vi "dfd_Convert Filter to String.vi"(5 "indent order":i32, 7 "format string":string="%-+022.16e", 11 "filter":T1={"mSRate_Fs"=1.0, "mSRate_Version"="1.0", "mSRate_Comments"="", "mSRate_OrgCoef"={"type"=enum."Undefined", "gain"=1.0, "coef a (k)"=[], "coef b (v)"=[]}, "mSRate_CurCoef"={"type"=enum."Undefined", "gain"=1.0, "coef a (k)"=[], "coef b (v)"=[]}, "mSRate_Quantized?"=FALSE, "mSRate_QCoef"={"type"=enum."Undefined", "gain"=1.0, "coef a (k)"=[], "coef b (v)"=[]}, "mSRate_QSettings"=[], "mSRate_Order"=0, "mSRate_Scaling"={"mSRate_ScaleByPowerOf2?"=FALSE, "mSRate_ScaleType"=enum."No Norm"}} {"mSRate_QSettings"."source" items=["Coef a/k"=0, "Coef b/v"=7, "Input"=1, "Output"=2, "Multiplicand"=3, "Product"=4, "Sum"=5, "Delay"=6, "Gain"=8]}) -> (3 "xml string":string)   [LabVIEW 2017, in "NI_DigFilter_Process.lvlib"]
uses:
  <vilib>/addons/Digital Filter Design/NI_DigFilter_Process.lvlib
  <vilib>/addons/Digital Filter Design/_Objects.llb/DFD Filter Obj.ctl
  <vilib>/addons/Digital Filter Design/_Objects.llb/DFD Filter Coef.ctl
  <vilib>/addons/Digital Filter Design/_Objects.llb/DFD Filter Structure Type Selector.ctl
  <vilib>/addons/Digital Filter Design/_Objects.llb/dfd_Internal Quantization Settings.ctl
  <vilib>/addons/Digital Filter Design/_Objects.llb/dfd_Internal Quantization Srcs.ctl
  <vilib>/addons/Digital Filter Design/_Objects.llb/DFD Coef Norm Type.ctl
  <vilib>/addons/Digital Filter Design/NI_DigFilterLicensed.lvlib
panel:
  in  "ZPK format string":string="%.16e"
  out "error out":errorcluster
  in  "error in (no error)":errorcluster
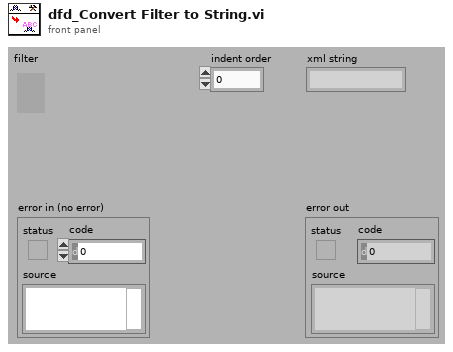
[diagram p1: front panel]
types:
  T1 = typedef "NI_DigFilterLicensed.lvlib/DFD Filter Obj.ctl" = cluster{"mSRate_Fs":dbl, "mSRate_Version":string, "mSRate_Comments":string, "mSRate_OrgCoef":T2, "mSRate_CurCoef":T2, "mSRate_Quantized?":bool, "mSRate_QCoef":T2, "mSRate_QSettings":T4[], "mSRate_Order":i32, "mSRate_Scaling":cluster{"mSRate_ScaleByPowerOf2?":bool, "mSRate_ScaleType":T6}}
  T2 = typedef "NI_DigFilterLicensed.lvlib/DFD Filter Coef.ctl" = cluster{"type":T3, "gain":dbl, "coef a (k)":dbl[], "coef b (v)":dbl[]}
  T3 = typedef "NI_DigFilterLicensed.lvlib/DFD Filter Structure Type Selector.ctl" = enum16{"Undefined", "FIR Direct Form", "FIR Direct Form Transposed", "FIR Symmetric", "FIR Antisymmetric", "IIR Direct Form I", "IIR Direct Form I Transposed", "IIR Direct Form II", "IIR Direct Form II Transposed", "IIR Cascaded Second Order Sections Form I", "IIR Cascaded Second Order Sections Form I Transposed", "IIR Cascaded Second Order Sections Form II", "IIR Cascaded Second Order Sections Form II Transposed", "Lattice Allpass (basic sections)", "Lattice Allpass (one multiplier sections)", "Lattice Allpass (normalized sections)", "Lattice AR (basic sections)", "Lattice AR (one multiplier sections)", "Lattice AR (normalized sections)", "Lattice MA (minimum phase)", "Lattice MA (maximum phase)", "Lattice ARMA (basic sections)", "Lattice ARMA (one multiplier sections)", "Lattice ARMA (normalized sections)"}
  T4 = typedef "NI_DigFilterLicensed.lvlib/dfd_Internal Quantization Settings.ctl" = cluster{"source":T5, "wl":i16, "iwl":i16, "overflow mode":enum16{"Saturation", "Wrap"}, "rounding mode":enum16{"Nearest", "Truncation"}, "signed?":bool}
  T5 = typedef "NI_DigFilterLicensed.lvlib/dfd_Internal Quantization Srcs.ctl" = u16
  T6 = typedef "NI_DigFilterLicensed.lvlib/DFD Coef Norm Type.ctl" = enum16{"No Norm", "Time Domain 1-Norm", "Time Domain 2-Norm", "Time Domain Inf-Norm"}
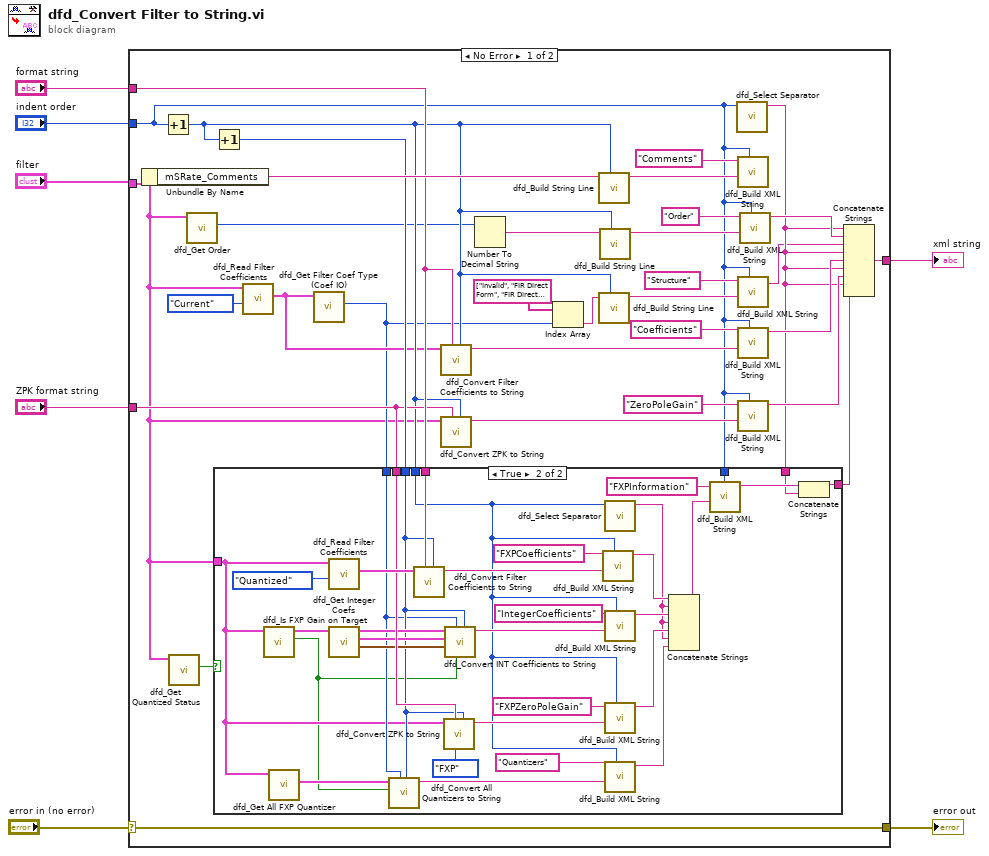
[diagram p0: block diagram]
diagram:
  n1 = case shown="No Error" "error in (no error)" {
    selector: "error in (no error)" -> [w31 w75]
    tunnel: "filter" -> [w10 _]
    tunnel: "format string" -> [w24 _]
    tunnel: [w32 _] -> w6
    tunnel: [w31 w75] -> w5
    tunnel: "indent order" -> [w16 _]
    tunnel: "ZPK format string" -> [w23 _]
    frame No Error {
      n2 = Unbundle By Name(w10) -> ("mSRate_Comments"=w29:string)
      n3 = Increment(x=w16) -> (x+1=w19:i32)
      n4 = call <vilib>:"dfd_Get Quantized Status.vi"("filter in"=w10) -> ("quantized?"=w26:bool)  [unwired: 1 in, 9 out]
      n5 = call <vilib>:"dfd_Get Order.vi"("filter in"=w10) -> ("order"=w11:i32)  [unwired: 1 in, 9 out]
      n6 = Increment(x=w19) -> (x+1=w25:i32)
      n7 = call <vilib>:"dfd_Read Filter Coefficients.vi"("coef source"=enum16{"Original", "Current", "Quantized"}."Current", "filter in"=w10) -> ("filter coef"=w14:T2)  [unwired: 1 in, 8 out]
      n8 = call <vilib>:"dfd_Get Filter Coef Type (Coef IO).vi"("filter coef in"=w14) -> ("type"=w12:T3)  [unwired: 1 in, 9 out]
      n9 = call <vilib>:"dfd_Convert Filter Coefficients to String.vi"("indent order"=w19, "format string"=w24, "filter coef"=w14) -> ("xml string out"=w38:string)  [unwired: 2 in, 6 out]
      n10 = call <vilib>:"dfd_Convert ZPK to String.vi"("indent order"=w19, "format string"=w23, "filter"=w10) -> ("xml string"=w30:string)  [unwired: 3 in, 5 out]
      n11 = Number To Decimal String(number=w11) -> (decimal integer string=w21:string)  [unwired: 1 out]
      n12 = Index Array(array=string[] ["Invalid", "FIR Direct Form", "FIR Direct Form Transposed", "FIR Symmetric", "FIR Antisymmetric", "IIR Direct Form I", "IIR Direct Form I Transposed", "IIR Direct Form II", "IIR Direct Form II Transposed", "IIR Cascaded Second-Order Sections Form I", "IIR Cascaded Second-Order Sections Form I Transposed", "IIR Cascaded Second-Order Sections Form II", "IIR Cascaded Second-Order Sections Form II Transposed", "Lattice Allpass (basic sections)", "Lattice Allpass (one multiplier sections)", "Lattice Allpass (normalized sections)", "Lattice AR (basic sections)", "Lattice AR (one multiplier sections)", "Lattice AR (normalized sections)", "Lattice MA (minimum phase)", "Lattice MA (maximum phase)", "Lattice ARMA (basic sections)", "Lattice ARMA (one multiplier sections)", "Lattice ARMA (normalized sections)"] ("Strings []"), index=w12) -> (element=w13:string)
      n13 = call <vilib>:"dfd_Build String Line.vi"("indent order"=w19, "string"=w29) -> ("string line"=w22:string)  [unwired: 9 out]
      n14 = call <vilib>:"dfd_Build String Line.vi"("indent order"=w19, "string"=w13) -> ("string line"=w28:string)  [unwired: 9 out]
      n15 = call <vilib>:"dfd_Build String Line.vi"("indent order"=w19, "string"=w21) -> ("string line"=w20:string)  [unwired: 9 out]
      n16 = call <vilib>:"dfd_Select Separator.vi"("indent order"=w16) -> ("separator"=w15:string)  [unwired: 10 out]
      n17 = case shown="True" w26 {
        tunnel: w10 -> [_ w43]
        tunnel: [_ w53] -> w33
        tunnel: w24 -> [_ w73]
        tunnel: w16 -> [_ w71]
        tunnel: w19 -> [_ w51]
        tunnel: w25 -> [_ w45]
        tunnel: w23 -> [_ w60]
        tunnel: w15 -> [_ w52]
        tunnel: w12 -> [_ w44]
        frame False {
        }
        frame True {
          n18 = call <vilib>:"dfd_Is FXP Gain on Target.vi"("filter in"=w43) -> ("Gain on Target?"=w42:bool, "dup filter out"=w41:T1)  [unwired: 9 out]
          n19 = call <vilib>:"dfd_Get All FXP Quantizer.vi"("filter in"=w43) -> ("quantization settings"=w46:T4[])  [unwired: 1 in, 9 out]
          n20 = call <vilib>:"dfd_Read Filter Coefficients.vi"("coef source"=enum16{"Original", "Current", "Quantized"}."Quantized", "filter in"=w43) -> ("filter coef"=w62:T2)  [unwired: 1 in, 8 out]
          n21 = call <vilib>:"dfd_Get Integer Coefs.vi"("filter"=w41) -> ("int gain"=w48:cluster{"wl":i16, "integer":i32}, "int coef a"=w49:cluster{"wl":i16, "integers":i32[]}, "int coef b"=w50:cluster{"wl":i16, "integers":i32[]})  [unwired: 1 in, 7 out]
          n22 = call <vilib>:"dfd_Convert All Quantizers to String.vi"("indent order"=w45, "filter type"=w44, "Gain on Target?"=w42, "quantization settings"=w46) -> ("string out"=w47:string)  [unwired: 7 out]
          n23 = call <vilib>:"dfd_Convert Filter Coefficients to String.vi"("indent order"=w45, "format string"=w73, "filter coef"=w62) -> ("xml string out"=w68:string)  [unwired: 2 in, 6 out]
          n24 = call <vilib>:"dfd_Convert ZPK to String.vi"("indent order"=w45, "type (FLP)"=enum16{"FLP", "FXP"}."FXP", "format string"=w60, "filter"=w43) -> ("xml string"=w58:string)  [unwired: 2 in, 5 out]
          n25 = call <vilib>:"dfd_Convert INT Coefficients to String.vi"("indent order"=w45, "Gain on Target?"=w42, "type"=w44, "int gain"=w48, "int coef a"=w49, "int coef b"=w50) -> ("xml string out"=w65:string)  [unwired: 1 in, 4 out]
          n26 = call <vilib>:"dfd_Build XML String.vi"("indent order"=w51, "string in"=w68, "element name"="FXPCoefficients") -> ("xml string out"=w67:string)  [unwired: 1 in, 7 out]
          n27 = call <vilib>:"dfd_Select Separator.vi"("indent order"=w51) -> ("separator"=w55:string)  [unwired: 10 out]
          n28 = call <vilib>:"dfd_Build XML String.vi"("indent order"=w51, "string in"=w65, "element name"="IntegerCoefficients") -> ("xml string out"=w63:string)  [unwired: 1 in, 7 out]
          n29 = call <vilib>:"dfd_Build XML String.vi"("indent order"=w51, "string in"=w58, "element name"="FXPZeroPoleGain") -> ("xml string out"=w61:string)  [unwired: 1 in, 7 out]
          n30 = call <vilib>:"dfd_Build XML String.vi"("indent order"=w51, "string in"=w47, "element name"="Quantizers") -> ("xml string out"=w57:string)  [unwired: 1 in, 7 out]
          n31 = Concatenate Strings(w67, w55, w63, w55, w61, w55, w57) -> (w66:string)
          n32 = call <vilib>:"dfd_Build XML String.vi"("indent order"=w71, "string in"=w66, "element name"="FXPInformation") -> ("xml string out"=w54:string)  [unwired: 1 in, 7 out]
          n33 = Concatenate Strings(w54, w52) -> (w53:string)
        }
      }
      n34 = call <vilib>:"dfd_Build XML String.vi"("indent order"=w16, "string in"=w22, "element name"="Comments") -> ()  [unwired: 2 in, 7 out]
      n35 = call <vilib>:"dfd_Build XML String.vi"("indent order"=w16, "string in"=w28, "element name"="Structure") -> ("xml string out"=w9:string)  [unwired: 1 in, 7 out]
      n36 = call <vilib>:"dfd_Build XML String.vi"("indent order"=w16, "string in"=w38, "element name"="Coefficients") -> ("xml string out"=w35:string)  [unwired: 1 in, 7 out]
      n37 = call <vilib>:"dfd_Build XML String.vi"("indent order"=w16, "string in"=w30, "element name"="ZeroPoleGain") -> ("xml string out"=w34:string)  [unwired: 1 in, 7 out]
      n38 = call <vilib>:"dfd_Build XML String.vi"("indent order"=w16, "string in"=w20, "element name"="Order") -> ("xml string out"=w17:string)  [unwired: 2 in, 6 out]
      n39 = Concatenate Strings(w15, w17, w9, w15, w35, w15, w34, w15, w33) -> (w32:string)
    }
    frame Error {
    }
  }
  "xml string" <- w6
  "error out" <- w5
